vi "fgv_overplot.vi"(0 "Data in":dbl[](array[numeric]), 2 "function (default: show)":enum16{"init", "add"}(ring), 7 "num for avg":u32, 9 "total samples":u32, 11 "error in":errorcluster) -> (4 "Plot":dbl[][](array[numeric]), 8 "SPC ALARM":bool, 15 "error out":errorcluster)   [LabVIEW 2022 SP3]
uses:
  <vilib>/Analysis/NI_AALBase.lvlib
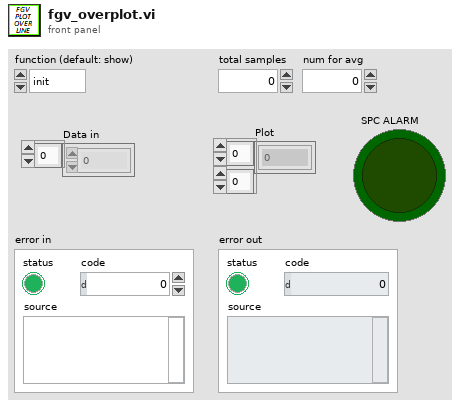
[diagram p1: front panel]
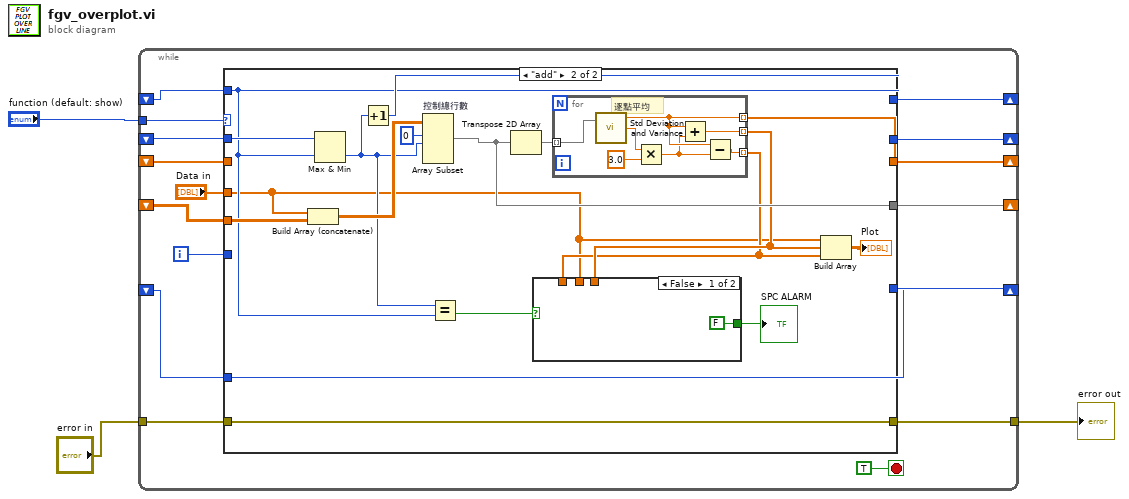
[diagram p0: block diagram]
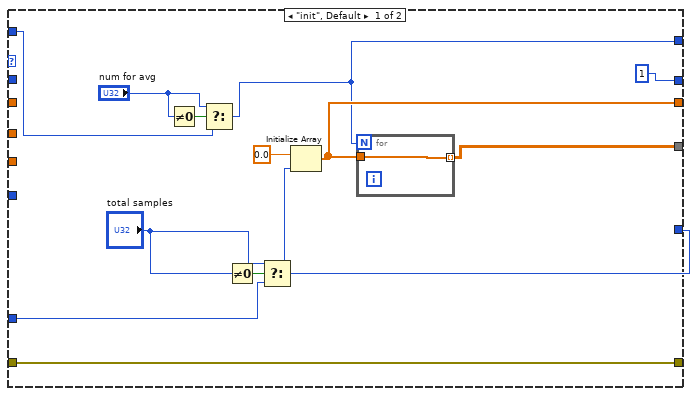
[diagram p2: hidden frame]
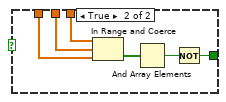
[diagram p3: hidden frame]
diagram:
  n1 = while {
    shift-right: [w18] -> _
    shift-left: _ -> [w17]
    tunnel: "function (default: show)" -> [w19]
    tunnel: [w15] -> w2
    tunnel: "error in" -> [w14]
    shift-right: [w13] -> _
    shift-left: _ -> [w12]
    shift-right: [w11] -> _
    shift-left: _ -> [w10]
    shift-right: [w9] -> _
    shift-left: _ -> [w8]
    shift-right: [w5] -> _
    shift-left: _ -> [w6]
    i -> [w7]
    stop <- TRUE stop-if-true
    n2 = case shown="\"add\"" w19 {
      tunnel: [w30 w43] -> w18
      tunnel: w17 -> [_ w48]
      tunnel: [w32 w50] -> w15
      tunnel: w14 -> [w32 w50]
      tunnel: [w29 w47] -> w13
      tunnel: w12 -> [_ _]
      tunnel: [w21 w37] -> w11
      tunnel: w10 -> [w23 w37]
      tunnel: [w25 w46] -> w9
      tunnel: w8 -> [w26 w46]
      tunnel: w7 -> [_ _]
      tunnel: w6 -> [_ w40]
      tunnel: [1 w39] -> w5
      tunnel: "Data in" -> [_ w34]
      frame "init", Default {
        n3 = Not Equal To 0?(x="num for avg") -> (x != 0?=w24:bool)
        n4 = Select(t="num for avg", s=w24, f=w23) -> (s? t:f=w21:u32)
        n5 = Not Equal To 0?(x="total samples") -> (x != 0?=w28:bool)
        n6 = Select(t="total samples", s=w28, f=w26) -> (s? t:f=w25:u32)
        n7 = Initialize Array(0.0 ("Numeric"), w25) -> (w29:dbl[])
        n8 = for {
          N: w21 -> [_]
          tunnel: [w33] -> w30 mode=indexing
          tunnel: w29 -> [w33]
        }
      }
      frame "add" {
        n9 = Build Array (concatenate)(w34, w48) -> (w45:dbl[][])
        n10 = Max & Min(x=w40, y=w37) -> (min(x,y)=w38:u32)  [unwired: 1 out]
        n11 = Increment(x=w38) -> (x+1=w39:u32)
        n12 = Array Subset "控制總行數"(array=w45, index (row)=0 ("index"), length (row)=w38) -> (w43:dbl[][])  [unwired: 2 in]
        n13 = Equal?(x=w38, y=w37) -> (x = y?=w35:bool)
        n14 = Transpose 2D Array(2D array=w43) -> (transposed array=w51:dbl[][])
        n15 = for {
          tunnel: w51 -> [w63] mode=indexing
          tunnel: [w62] -> w47 mode=indexing
          tunnel: [w60] -> w42 mode=indexing
          tunnel: [w59] -> w41 mode=indexing
          # "逐點平均"
          n16 = call <vilib>:"Std Deviation and Variance.vi"("X"=w63) -> ("mean"=w62:dbl, "standard deviation"=w65:dbl)  [unwired: 1 in, 1 out]
          n17 = Multiply(x=w65, y=3.0) -> (x*y=w61:dbl)
          n18 = Add(x=w62, y=w61) -> (x+y=w60:dbl)
          n19 = Subtract(x=w62, y=w61) -> (x-y=w59:dbl)
        }
        n20 = case shown="False" w35 {
          tunnel: w34 -> [_ w58]
          tunnel: w42 -> [_ w57]
          tunnel: w41 -> [_ w56]
          tunnel: [FALSE w53] -> w36
          frame False {
          }
          frame True {
            n21 = In Range and Coerce(upper limit=w57, x=w58, lower limit=w56) -> (In Range?=w55:bool[])  [unwired: 1 out]
            n22 = And Array Elements(Boolean array=w55) -> (logical AND=w54:bool)
            n23 = Not(x=w54) -> (.not. x?=w53:bool)
          }
        }
        "SPC ALARM" <- w36
        n24 = Build Array(w34, w42, w41) -> (→"Plot":dbl[][])
      }
    }
  }
  "error out" <- w2
